vi "5492_TaylorSeriesNaturalLog.vi"(10 "x":dbl format="%#_13g") -> (2 "ln(x)":dbl format="%#_13g")   [LabVIEW 2016]
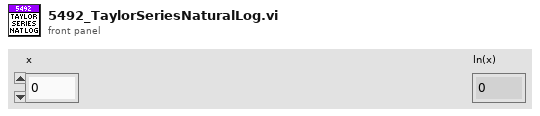
[diagram p1: front panel]
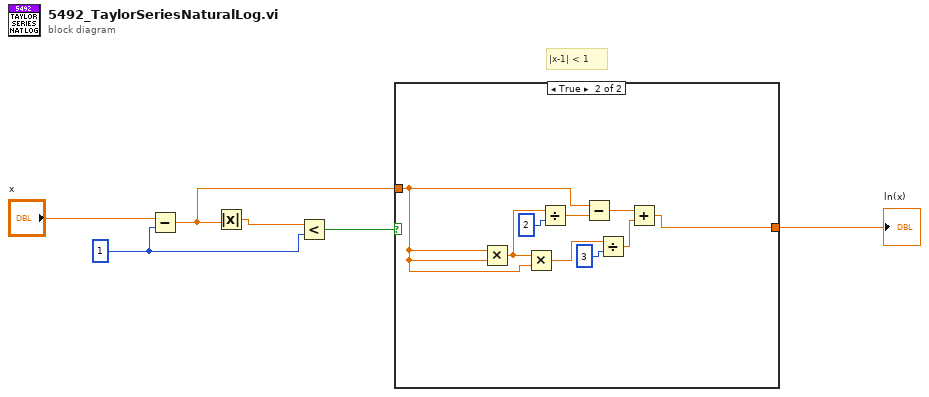
[diagram p0: block diagram]
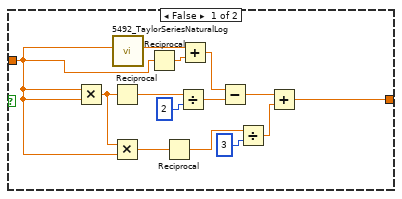
[diagram p2: hidden frame]
diagram:
  w5 = 1
  # "|x-1| < 1"
  n1 = Subtract(x="x", y=w5) -> (x-y=w2:dbl)
  n2 = Absolute Value(x=w2) -> (abs(x)=w6:dbl)
  n3 = Less?(x=w6, y=w5) -> (x < y?=w4:bool)
  n4 = case shown="True" w4 {
    tunnel: w2 -> [w13 w24]
    tunnel: [w7 w25] -> w1
    frame False {
      n5 = Multiply(x=w13, y=w13) -> (x*y=w14:dbl)
      n6 = Reciprocal(x=w14) -> (1/x=w16:dbl)
      n7 = Multiply(x=w14, y=w13) -> (x*y=w12:dbl)
      n8 = call "5492_TaylorSeriesNaturalLog.vi"("x"=w13) -> ("ln(x)"=w20:dbl)  [unwired: 10 in]
      n9 = Reciprocal(x=w13) -> (1/x=w19:dbl)
      n10 = Reciprocal(x=w12) -> (1/x=w11:dbl)
      n11 = Divide(x=w16, y=2) -> (x/y=w17:dbl)
      n12 = Add(x=w20, y=w19) -> (x+y=w18:dbl)
      n13 = Subtract(x=w18, y=w17) -> (x-y=w8:dbl)
      n14 = Divide(x=w11, y=3) -> (x/y=w9:dbl)
      n15 = Add(x=w8, y=w9) -> (x+y=w7:dbl)
    }
    frame True {
      n16 = Multiply(x=w24, y=w24) -> (x*y=w22:dbl)
      n17 = Multiply(x=w22, y=w24) -> (x*y=w23:dbl)
      n18 = Divide(x=w22, y=2) -> (x/y=w28:dbl)
      n19 = Subtract(x=w24, y=w28) -> (x-y=w27:dbl)
      n20 = Divide(x=w23, y=3) -> (x/y=w26:dbl)
      n21 = Add(x=w27, y=w26) -> (x+y=w25:dbl)
    }
  }
  "ln(x)" <- w1
